vi "gui binning.vi"(8 "error in (no error)":errorcluster, 11 "Point Grey Camera in":refnum<class "Point Grey Camera.lvclass">) -> (0 "error out":errorcluster)   [LabVIEW 2020, in "Point Grey Camera.lvclass"]
uses:
  Point Grey Camera.lvclass
  Point Grey Camera.lvclass/Point Grey Camera.ctl
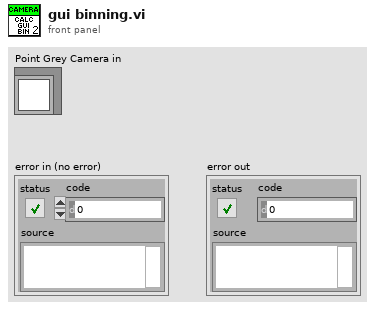
[diagram p1: front panel]
types:
  T1 = typedef "IMAQ Image.ctl" = refnum<image>
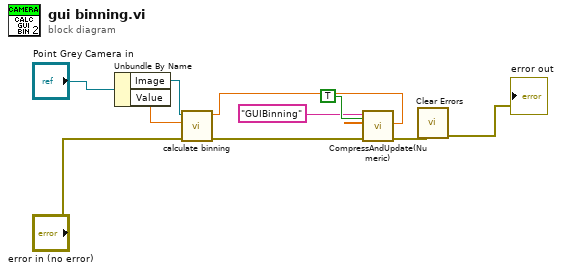
[diagram p0: block diagram]
diagram:
  n1 = Unbundle By Name("Point Grey Camera in") -> ("Image"=w9:T1, "Value"=w10:dbl)
  n2 = call "calculate binning.vi"("error in (no error)"="error in (no error)", "MaxGuiPixel"=w10, "Refnum in"=w9) -> ("error out"=w7:errorcluster, "GUIbinning"=w2:dbl)  [unwired: 7 in]
  n3 = call "CompressAndUpdate(Numeric).vi"("force CVT update (false)"=TRUE, "error in"=w7, "Numeric"=w2, "command or variable name"="GUIBinning") -> ("error out"=w8:errorcluster)  [unwired: 7 in]
  n4 = call "Clear Errors.vi"("error in (no error)"=w8) -> ("error out"=→"error out":errorcluster)  [unwired: 5 in, 1 out]
